vi "Read Digital Port.vi"(8 "error in (no error)":errorcluster, 11 "NI Digital Input":refnum<class "NI DIO.lvclass">) -> (0 "error out":errorcluster, 2 "DIs":bool[](array[boolean]), 3 "NI Digital Input out":refnum<class "NI DIO.lvclass">)   [LabVIEW 2025, in "Digital IO.lvlib" / "NI DIO.lvclass"]
uses:
  NI DIO.lvclass
  NI DIO.lvclass/NI DIO.ctl
  <vilib>/DAQmx/read.llb/DAQmx Read (Digital 1D Bool NChan 1Samp 1Line).vi
  <vilib>/DAQmx/miscellaneous.llb/DAQmx Fill In Error Info.vi
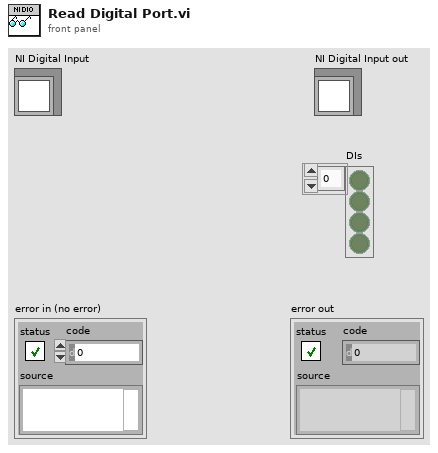
[diagram p1: front panel]
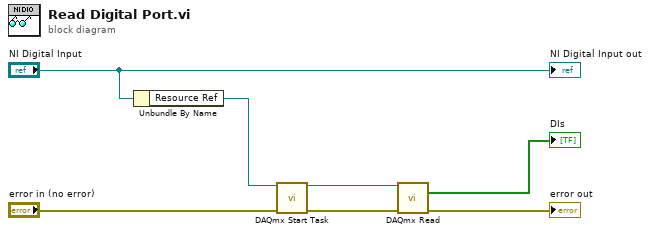
[diagram p0: block diagram]
diagram:
  n1 = Unbundle By Name("NI Digital Input") -> ("Resource Ref"=w4:refnum<k21>)
  n2 = call <vilib>:"DAQmx Start Task.vi"("task/channels in"=w4, "error in"="error in (no error)") -> ("task out"=w1:refnum<k21>, "error out"=w2:errorcluster)  [unwired: 12 in]
  n3 = call-poly <vilib>:"DAQmx Read.vi"("task/channels in"=w1, "error in"=w2) -> ("data"=→"DIs":bool[], "error out"=→"error out":errorcluster)  [unwired: 11 in, 1 out]
  "NI Digital Input out" <- "NI Digital Input"
